vi "Menu Resolve Source Str.vi"(0 "字符串":string) -> (1 "菜单信息":cluster{"父菜单名":string, "菜单项":string[]}[](array[cluster]), 2 "菜单详情":T2(array[cluster]))   [LabVIEW 2011]
uses:
  <vilib>/Utility/miscctls.llb/LVMenuShortCut.ctl
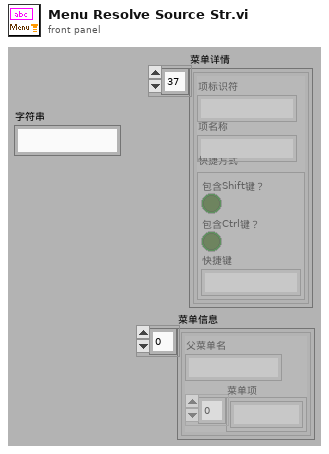
[diagram p1: front panel]
types:
  T1 = typedef "LVMenuShortCut.ctl" = cluster{"Include Shift Key?":bool, "Include Ctrl Key?":bool, "Shortcut Key":string}
  T2 = cluster{"项标识符":string, "项名称":string, "快捷方式":T1}[]
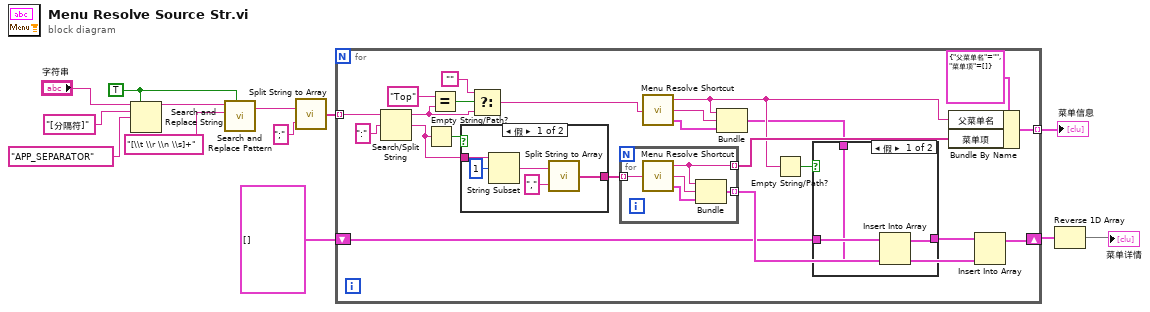
[diagram p0: block diagram]
diagram:
  w3 = TRUE ("替换全部？(F)")
  n1 = Search and Replace String(replace all?=w3, input string="字符串", search string="[分隔符]" ("搜索字符串"), replace string="APP_SEPARATOR" ("替换字符串(\"\")")) -> (result string=w4:string)  [unwired: 1 in, 6 out]
  n2 = call <vilib>:"Search and Replace Pattern.vi"("string"=w4, "regular expression (\"\")"="[\\t \\r \\n \\s]+" ("regular expression (\"\")"), "replace all? (F)"=w3) -> ("result string"=w2:string)  [unwired: 2 in, 1 out]
  n3 = call "Split String to Array.vi"("搜索字符串/字符(-)"=";", "字符串"=w2) -> ("字符串数组"=w13:string[])
  n4 = for {
    tunnel: w13 -> [w35] mode=indexing
    tunnel: [w26] -> w12 mode=indexing
    shift-right: [w14] -> w6
    shift-left: T2 [] -> [w16]
    n5 = Search/Split String(string=w35, search string/char (-)=":" ("搜索字符串/字符(-)")) -> (substring before match=w31:string, match + rest of string=w28:string)  [unwired: 2 out]
    n6 = Empty String/Path?(string/path=w28) -> (empty?=w29:bool)
    n7 = Equal?(x="Top", y=w31) -> (x = y?=w32:bool)
    n8 = case shown="假" w29 {
      tunnel: w28 -> [w49 _]
      tunnel: [w45 _] -> w24
      frame False {
        n9 = String Subset(string=w49, offset (0)=1 ("偏移量(0)")) -> (substring=w47:string)  [unwired: 1 out]
        n10 = call "Split String to Array.vi"("搜索字符串/字符(-)"=",", "字符串"=w47) -> ("字符串数组"=w45:string[])
      }
      frame True {
      }
    }
    n11 = Select(t="", s=w32, f=w31) -> (s? t:f=w25:string)
    n12 = for {
      tunnel: w24 -> [w44] mode=indexing
      tunnel: [w43] -> w23 mode=indexing
      tunnel: [w40] -> w17 mode=indexing
      n13 = call "Menu Resolve Shortcut.vi"("输入字符串"=w44) -> ("快捷方式"=w41:T1, "项名称"=w42:string, "项标识符"=w43:string)
      n14 = Bundle("项标识符"=w43, "项名称"=w42, "快捷方式"=w41) -> (w40:cluster{"项标识符":string, "项名称":string, "快捷方式":T1})  [unwired: 1 in]
    }
    n15 = call "Menu Resolve Shortcut.vi"("输入字符串"=w25) -> ("快捷方式"=w19:T1, "项名称"=w20:string, "项标识符"=w21:string)
    n16 = Bundle("项标识符"=w21, "项名称"=w20, "快捷方式"=w19) -> (w18:cluster{"项标识符":string, "项名称":string, "快捷方式":T1})  [unwired: 1 in]
    n17 = Empty String/Path?(string/path=w21) -> (empty?=w22:bool)
    n18 = case shown="假" w22 {
      tunnel: w18 -> [w37 _]
      tunnel: w16 -> [w38 w39]
      tunnel: [w36 w39] -> w15
      frame False {
        n19 = Insert Into Array(array=w38, new element=w37) -> (w36:T2)  [unwired: 1 in]
      }
      frame True {
      }
    }
    n20 = Bundle By Name(cluster=cluster{"父菜单名":string, "菜单项":string[]} {"父菜单名"="", "菜单项"=[]} ("菜单项"), "父菜单名"=w21, "菜单项"=w23) -> (w26:cluster{"父菜单名":string, "菜单项":string[]})
    n21 = Insert Into Array(array=w15, new element=w17) -> (w14:T2)  [unwired: 1 in]
  }
  "菜单信息" <- w12
  n22 = Reverse 1D Array(array=w6) -> (reversed array=→"菜单详情":T2)
